vi "test - Unregister Status Registration.vi"(8 "error in (no error)":errorcluster, 11 "TestCase in":refnum<class "testcase-Broadcast Registry.lvclass">) -> (0 "error out":errorcluster, 3 "TestCase out":refnum<class "testcase-Broadcast Registry.lvclass">)   [LabVIEW 2017, in "testcase-Broadcast Registry.lvclass"]
uses:
  testcase-Broadcast Registry.lvclass
  f1ab6f25-c30d-499f-96ca-3a55fa643449.vi
  src/user.lib/_NEVSTOP/Communicable State Machine(CSM)/AdvanceAPI/CSM - Revert Arguments-Safe String.vi
  src/user.lib/_NEVSTOP/Communicable State Machine(CSM)/AdvanceAPI/CSM - Make String Arguments Safe.vi
  src/user.lib/_NEVSTOP/Communicable State Machine(CSM)/AdvanceAPI/CSM - Break Down Multiple States String.vi
  src/user.lib/_NEVSTOP/Communicable State Machine(CSM)/AdvanceAPI/CSM - Compact Multiple States.vi
  src/user.lib/_NEVSTOP/Communicable State Machine(CSM)/AdvanceAPI/CSM - Keywords.vi
  src/user.lib/_NEVSTOP/Communicable State Machine(CSM)/_Shared/Trim Single-line Text.vi
  <vilib>/addons/_JKI Toolkits/VI Tester/TestCase.llb/TestCase.lvclass
  src/user.lib/_NEVSTOP/Communicable State Machine(CSM)/Communicable State Machine.lvlib
  C:/Program Files (x86)/National Instruments/LabVIEW 2017/vi.lib/addons/_JKI Toolkits/VI Tester/TestCase.llb/TestCase.lvclass
panel:
  out "Entries":T1(array[cluster])
  out "Error Occurred":errorcluster
  out "State History":string
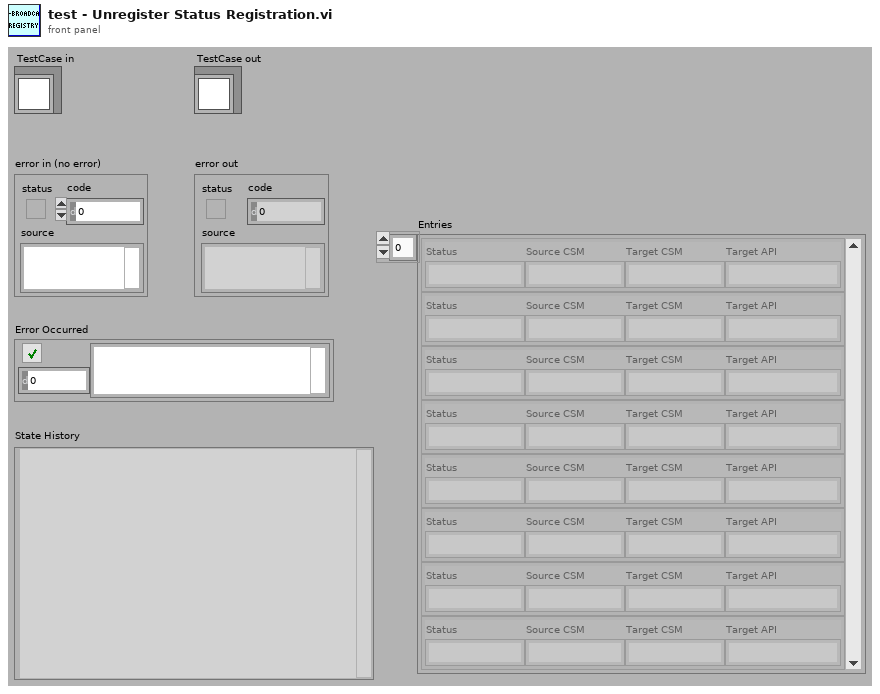
[diagram p1: front panel]
types:
  T1 = cluster{"Status":string, "Source CSM":string, "Target CSM":string, "Target API":string}[]
  T2 = enum32{"Invalid", "Standard", "Closed", "Hidden", "Minimized", "Maximized"}
  T3 = enum32{"invalid app kind", "Development System", "Run Time System", "Student Edition", "Embedded LabVIEW", "Evaluation", "Custom"}
  T4 = typedef "Communicable State Machine.lvlib/_CSM_Response Source Message.ctl" = cluster{"‘State":string, "’Arguments":string, "’Error":errorcluster}
  T5 = cluster{"Current VI Reference":refnum<vi>, "Close Panel on Exit?":bool}
  T6 = cluster{"Core":cluster{"Current VI Reference":refnum<vi>, "Close Panel on Exit?":bool}, "Your Boolean data":bool, "Your string data":string}
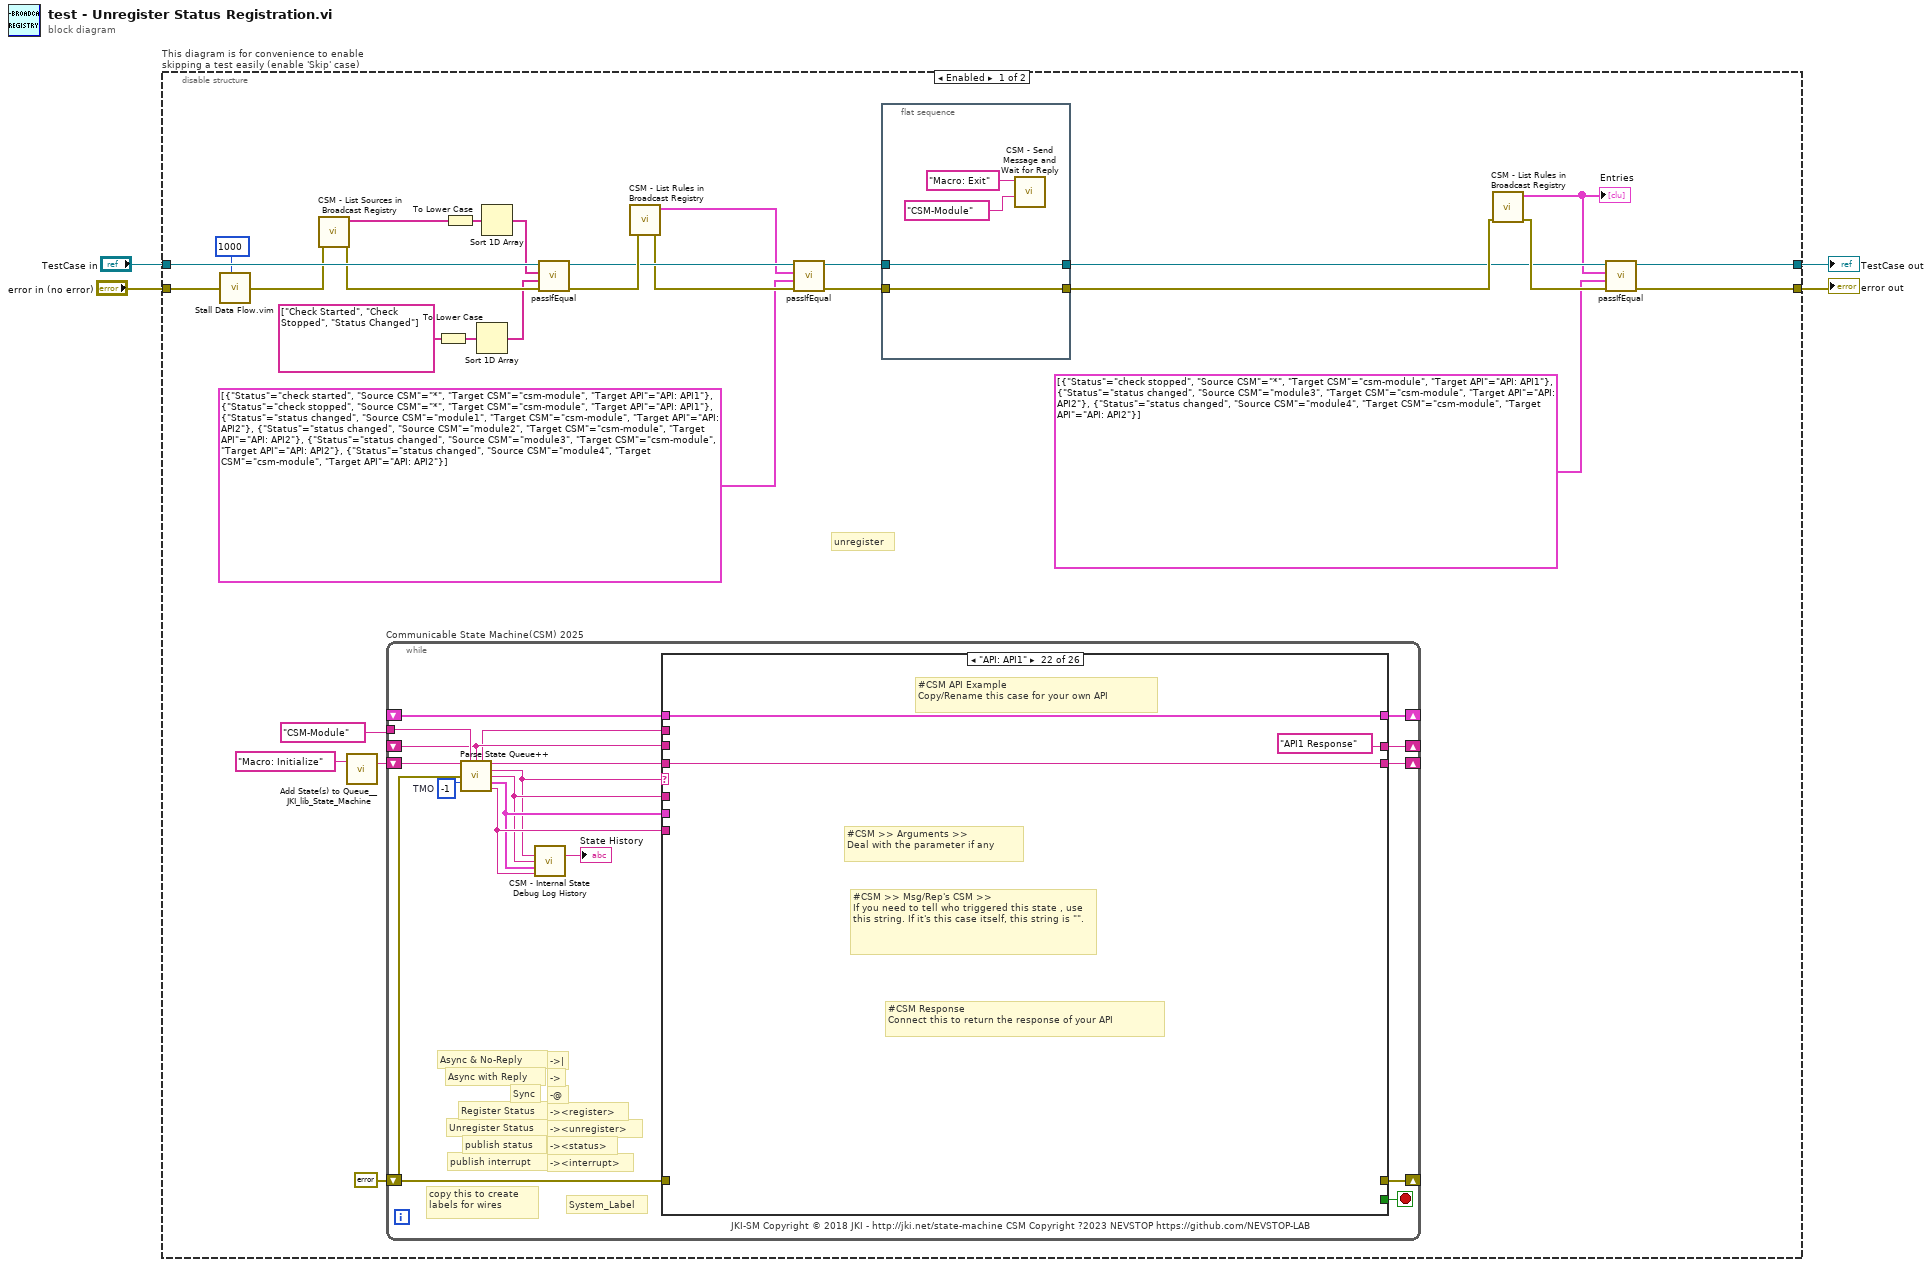
[diagram p0: block diagram]
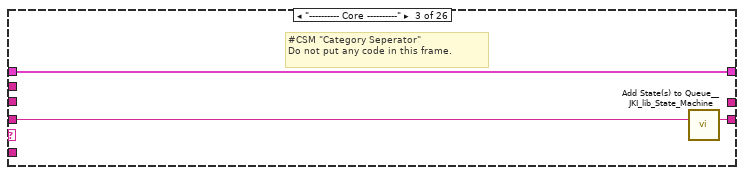
[diagram p4: hidden frame]
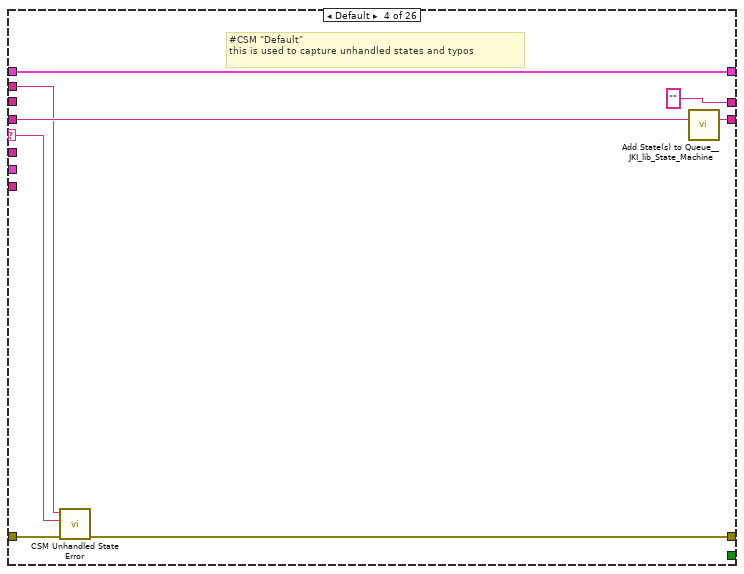
[diagram p5: hidden frame]
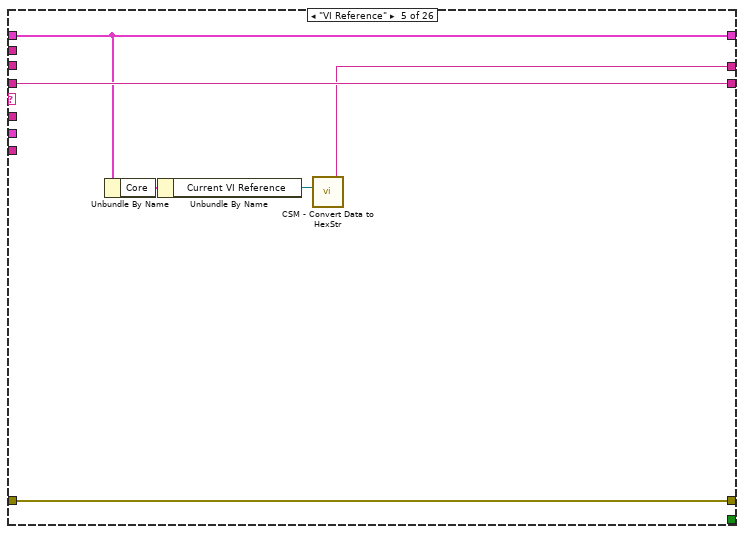
[diagram p6: hidden frame]
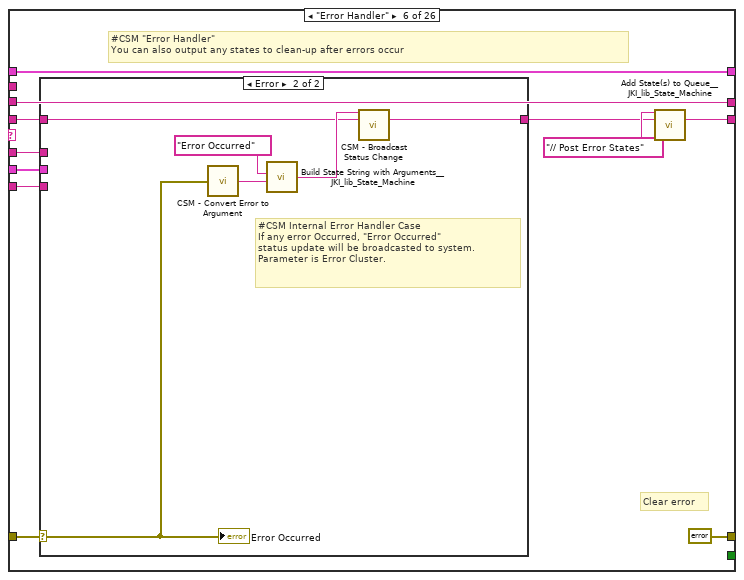
[diagram p7: hidden frame]
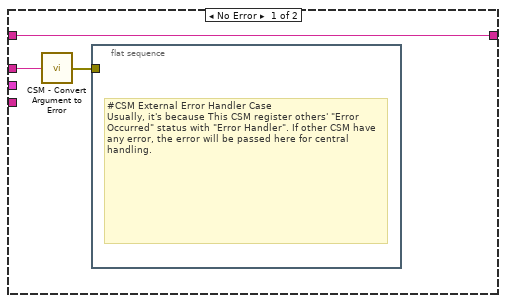
[diagram p8: hidden frame]
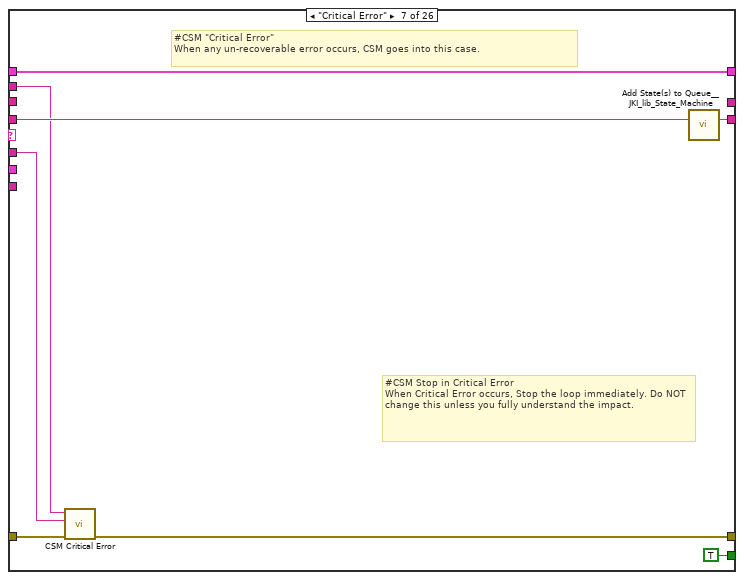
[diagram p9: hidden frame]
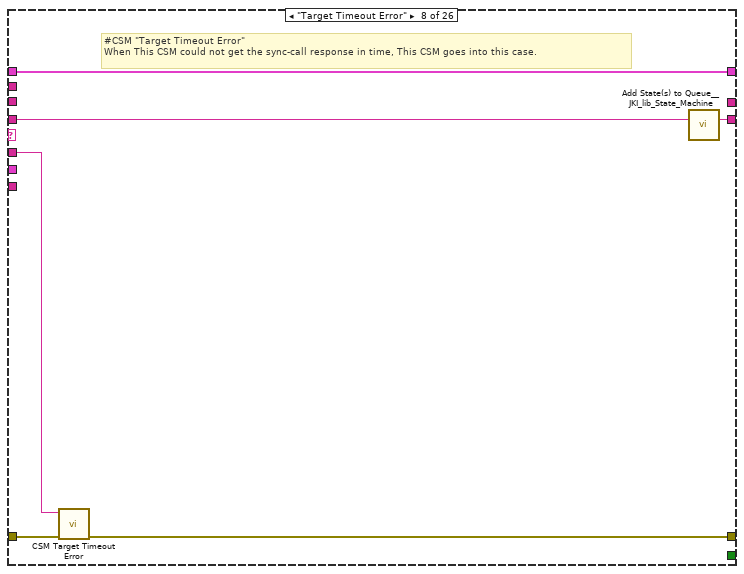
[diagram p10: hidden frame]
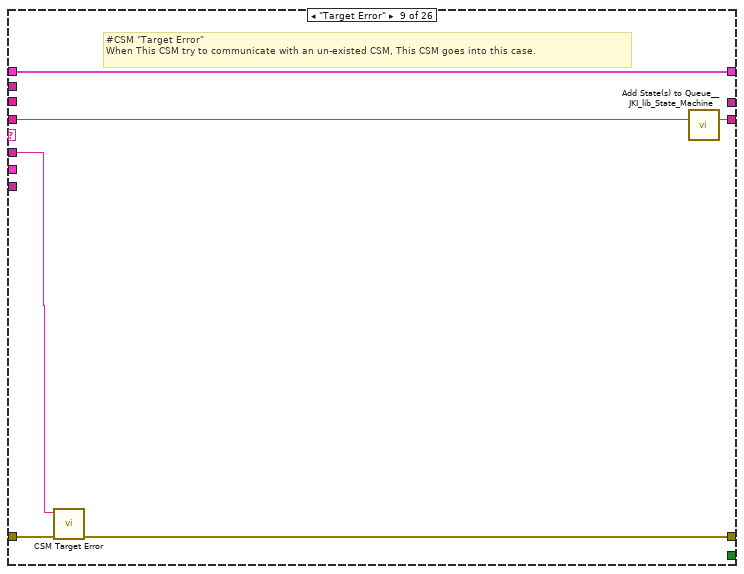
[diagram p11: hidden frame]
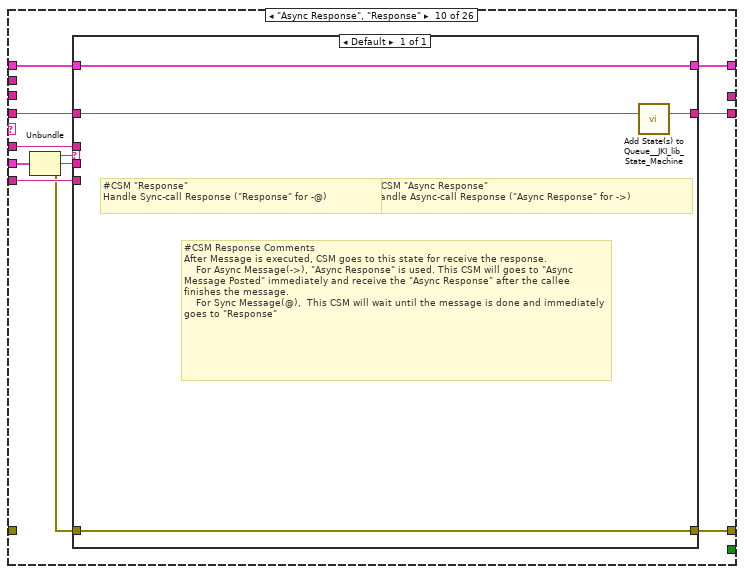
[diagram p12: hidden frame]
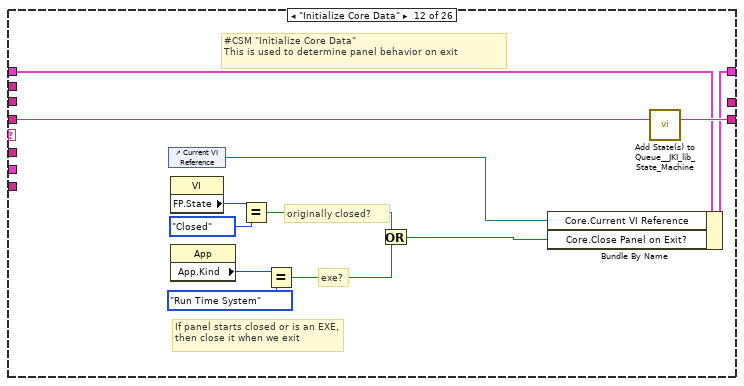
[diagram p14: hidden frame]
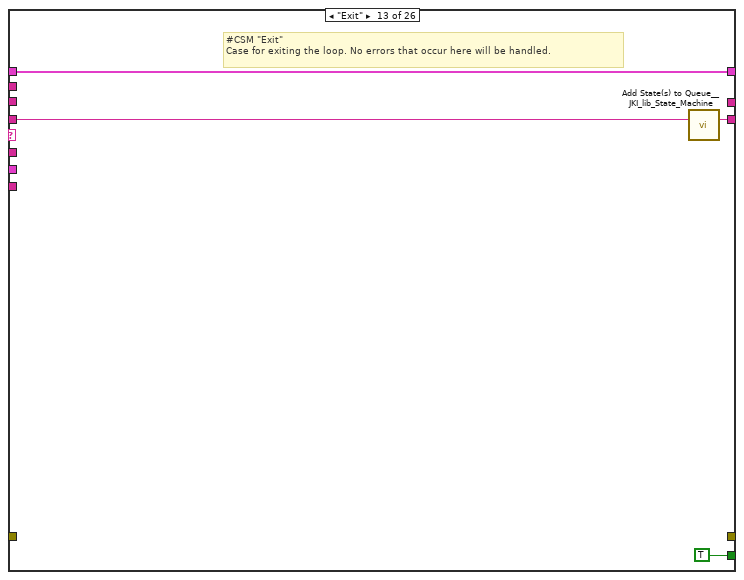
[diagram p15: hidden frame]
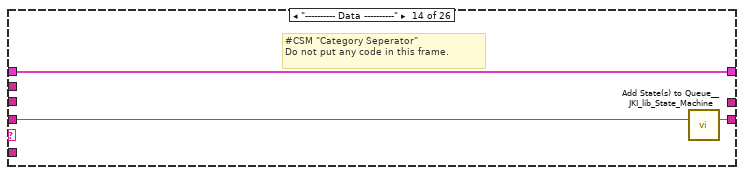
[diagram p16: hidden frame]
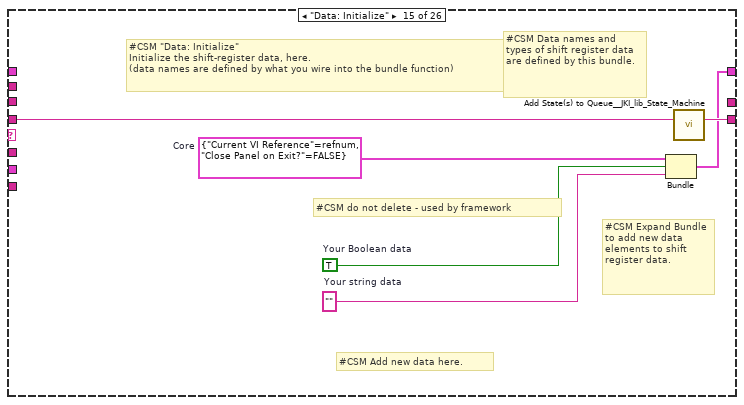
[diagram p17: hidden frame]
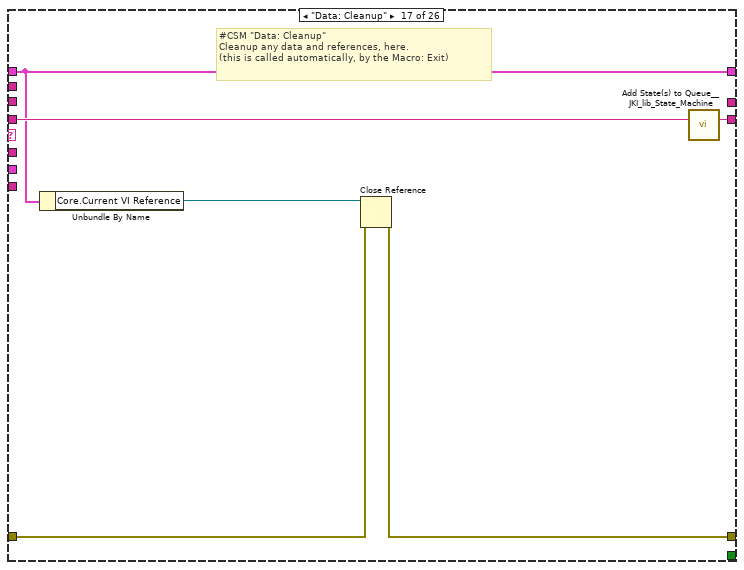
[diagram p19: hidden frame]
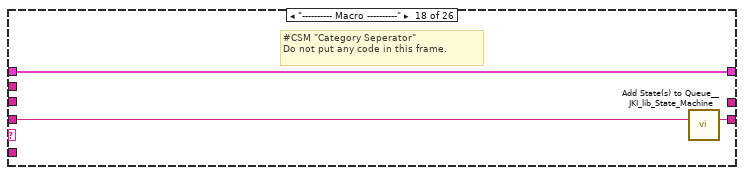
[diagram p20: hidden frame]
diagram:
  n1 = disable-structure "This diagram is for convenience to enable skipping a test easily (enable 'Skip' case)" shown="Enabled" {
    disable-tunnel: "TestCase in" -> [w33 w203]
    disable-tunnel: [w8 w201] -> w1
    disable-tunnel: [w7 w202] -> w3
    disable-tunnel: "error in (no error)" -> [w32 w200]
    frame Enabled {
      # "unregister"
      n2 = call "Stall Data Flow.vim"("value in"=w32, "milliseconds to wait"=u32 1000) -> ("value out"=w27:errorcluster)  [unwired: 1 out]
      n3 = call "CSM - List Sources in Broadcast Registry.vi"("error in (no error)"=w27) -> ("error out"=w25:errorcluster, "Broadcast Names"=w24:string[])  [unwired: 9 in]
      n4 = call <vilib>:"Add State(s) to Queue__JKI_lib_State_Machine.vi"("State(s) in (\"\")"="Macro: Initialize" ("Init State(\"Macro: Initialize\")")) -> ("States Out"=w31:string)  [unwired: 14 in]
      n5 = while "Communicable State Machine(CSM) 2025" {
        shift-right: [w50] -> _
        shift-left: _ -> [w49]
        shift-right: [w53] -> _
        shift-left: errorcluster {"status"=FALSE, "code"=0, "source"=""} ("error out") -> [w39]
        shift-right: [w52] -> _
        shift-left: w31 -> [w54]
        tunnel: "CSM-Module" ("Name (\"\" to Use UUID)") -> [w46]
        shift-right: [w47] -> _
        shift-left: _ -> [w41]
        stop <- w51 stop-if-true
        w48 = -1  # TMO
        # "-><interrupt>"
        # "-><status>"
        # "-><unregister>"
        # "-><register>"
        # "-@"
        # "->"
        # "->|"
        # "publish interrupt"
        # "publish status"
        # "Unregister Status"
        # "Register Status"
        # "Sync"
        # "Async with Reply"
        # "Async & No-Reply"
        # "JKI-SM Copyright © 2018 JKI - http://jki.net/state-machine CSM Copyright ?2023 NEVSTOP https://github.com/NEVSTOP-LAB"
        # "copy this to create labels for wires"
        # "System_Label"
        n6 = call "Parse State Queue++.vi"("State Queue"=w54, "Name (\"\" to Use UUID)"=w46, "Response Arguments"=w41, "Previous Error"=w39, "Dequeue (1 ms)"=w48) -> ("Name Used"=w40:string, "Remaining States"=w55:string, "Current State"=w42:string, "Arguments"=w43:string, "Additional Information"=w44:T4, "Source CSM"=w45:string)  [unwired: 5 in]
        n7 = call "CSM - Internal State Debug Log History.vi"("State"=w42, "Arguments (\"\")"=w43, ">> Response Source Message >>"=w44, "Source (\"\")"=w45) -> ("Debug Log"=→"State History":string)  [unwired: 11 in]
        n8 = case shown="\"API: API1\"" w42 {
          selector: w42 -> [_ _ _ w66 _ _ _ _ _ _ _ _ _ _ _ _ _ _ _ _ _ _ _ _ _ _]
          tunnel: w55 -> [w56 w59 w62 w70 w75 w81 w104 w110 w116 w126 w133 w145 w149 w152 w158 w160 w166 w169 w173 w179 w181 w184 w188 w193 w196 w199]
          tunnel: w43 -> [_ _ _ _ _ w80 w100 w107 w113 w120 _ _ _ _ _ _ _ _ _ _ _ _ w186 _ _ _]
          tunnel: w49 -> [w57 w58 w60 w68 w74 w86 w102 w108 w114 w124 w132 w139 w147 w150 _ w159 w161 w167 w171 w177 w180 w183 w187 w191 w194 w197]
          tunnel: [_ _ _ w63 w76 errorcluster {"status"=FALSE, "code"=0, "source"=""} ("error out") w97 w105 w111 w127 _ _ _ _ _ _ w162 _ _ _ _ _ _ _ _ _] -> w53
          tunnel: w39 -> [_ _ _ w64 w76 w84 w98 w106 w112 _ _ _ _ _ _ _ w163 _ _ _ _ _ _ _ _ _]
          tunnel: [w56 w59 w61 w69 w75 w82 w103 w109 w115 w125 w133 w144 w148 w151 w157 w160 w165 w168 w172 w178 w181 w184 w188 w192 w195 w198] -> w52
          tunnel: [_ _ _ _ _ _ TRUE _ _ _ _ _ TRUE _ _ _ _ _ _ _ _ _ _ _ _ _] -> w51
          tunnel: [w57 w58 w60 w68 w74 w86 w102 w108 w114 w123 w132 w143 w147 w150 w156 w159 w161 w167 w171 w177 w180 w183 w187 w191 w194 w197] -> w50
          tunnel: w45 -> [_ _ _ _ _ w79 _ _ _ w121 _ _ _ _ _ _ _ _ _ _ _ _ _ _ _ _]
          tunnel: w44 -> [_ _ _ _ _ w78 _ _ _ w122 _ _ _ _ _ _ _ _ _ _ _ _ _ _ _ _]
          tunnel: [_ _ _ "" w71 w77 _ _ _ _ _ _ _ _ _ _ _ _ _ _ _ "API1 Response" w185 _ _ _] -> w47
          tunnel: w40 -> [_ _ _ w65 _ _ w99 _ _ _ _ _ _ _ _ _ _ _ _ _ _ _ _ _ _ _]
          tunnel: w41 -> [_ _ _ _ _ w77 _ _ _ _ _ _ _ _ _ _ _ _ _ _ _ _ _ _ _ _]
          frame "", "Idle" {
            # "#CSM \"Idle/Event Handler\"\nexecutes when the state queue is empty"
          }
          frame "CSM Documentation" {
            # "#CSM Documentation"
            # "#CSM State Syntax\n\n// Comment line, all text to the right of “//” will be ignored\n// Local Message Example\nDoSth: DoA >> Arguments\n\n// Sync Call Example\nAPI: xxxx >> Arguments -@ TargetModule\n\n// Async Call Example\nAPI: xxxx >> Arguments -> TargetModule\n\n// Async Call without Reply Example\nAPI: xxxx >> Arguments ->| TargetModule\n\n// Broadcast normal status:\nStatus >> StatusArguments  -><status>\n\n// Broadcast Interrupt status:\nInterrupt >> StatusArguments  -><interrupt>\n\n// Register Source Module's status to Handler Module\nStatus@Source Module >> Handler Module@Handler Module -><register>\n\n// Unegister Source Module's status\nStatus@Source Module >> Handler Module -><unregister>"
            # "#CSM README FIRST\n\nCommunicable State Machine(CSM) is a LabVIEW application framework that builds upon JKI State Machine(JKISM). It follows the pattern of JKISM and extends the keywords to describe message communication between modules, including concepts such as Sync-Message, Async-Message, Subscription/Unsubscription of status - essential elements for creating reusable code modules. For more information, please visit the CSM wiki: https://nevstop-lab.github.io/CSM-Wiki/\n\nFor instructions on JKI State Machine, visit: \n    http://jki.net/state-machine/\nFor information about CSM, visit: \n    https://github.com/NEVSTOP-LAB"
            # "#CSM \"Documentation\"\nCase for holding CSM Documenation"
          }
          frame "---------- Core ----------" {
            # "#CSM \"Category Seperator\"\nDo not put any code in this frame."
            n9 = call <vilib>:"Add State(s) to Queue__JKI_lib_State_Machine.vi"("State(s) in (\"\")"=w62) -> ("States Out"=w61:string)  [unwired: 14 in]
          }
          frame Default {
            # "#CSM \"Default\"\nthis is used to capture unhandled states and typos"
            n10 = call "CSM Unhandled State Error.vi"("error in (no error)"=w64, "Undefined State"=w66, "CSM Name"=w65) -> ("error out"=w63:errorcluster)  [unwired: 8 in]
            n11 = call <vilib>:"Add State(s) to Queue__JKI_lib_State_Machine.vi"("State(s) in (\"\")"=w70) -> ("States Out"=w69:string)  [unwired: 14 in]
          }
          frame "VI Reference" {
            n12 = Unbundle By Name(w74) -> ("Core"=w73:T5)
            n13 = Unbundle By Name(w73) -> ("Current VI Reference"=w72:refnum<vi>)
            n14 = call "CSM - Convert Data to HexStr.vi"("Variant"=w72) -> ("HEX String (0-9,A-F)"=w71:string)  [unwired: 8 in]
          }
          frame "Error Handler" {
            # "#CSM \"Error Handler\"\nYou can also output any states to clean-up after errors occur"
            # "Clear error"
            n15 = case shown="Error" w84 {
              selector: w84 -> [_ w91]
              tunnel: [w90 w93] -> w83
              tunnel: w81 -> [w90 w92]
              tunnel: w80 -> [w89 _]
              tunnel: w79 -> [_ _]
              tunnel: w78 -> [_ _]
              frame No Error {
                n16 = call "CSM - Convert Argument to Error.vi"("Argument"=w89) -> ("Error"=w88:errorcluster)  [unwired: 4 in]
                n17 = flat-sequence {
                  tunnel: w88 -> [_]
                  frame #0 {
                    # "#CSM External Error Handler Case\nUsually, it's because This CSM register others' \"Error Occurred\" status with \"Error Handler\". If other CSM have any error, the error will be passed here for central handling."
                  }
                }
              }
              frame Error {
                # "#CSM Internal Error Handler Case \nIf any error Occurred, \"Error Occurred\" \nstatus update will be broadcasted to system.\nParameter is Error Cluster."
                n18 = call "CSM - Convert Error to Argument.vi"("Error"=w91) -> ("Argument"=w95:string)  [unwired: 4 in]
                n19 = call <vilib>:"Build State String with Arguments__JKI_lib_State_Machine.vi"("Arguments (\"\")"=w95, "State"="Error Occurred" ("Status with Arguments")) -> ("State with Arguments"=w94:string)  [unwired: 4 in]
                n20 = call "CSM - Broadcast Status Change.vi"("Status With Arguments"=w94, "State Queue"=w92) -> ("Remaining States"=w93:string)  [unwired: 13 in]
                "Error Occurred" <- w91
              }
            }
            n21 = call <vilib>:"Add State(s) to Queue__JKI_lib_State_Machine.vi"("State(s) in Front (\"\")"="// Post Error States", "State(s) in (\"\")"=w83) -> ("States Out"=w82:string)  [unwired: 13 in]
          }
          frame "Critical Error" {
            # "#CSM \"Critical Error\"\nWhen any un-recoverable error occurs, CSM goes into this case."
            # "#CSM Stop in Critical Error\nWhen Critical Error occurs, Stop the loop immediately. Do NOT change this unless you fully understand the impact."
            n22 = call "CSM Critical Error.vi"("error in (no error)"=w98, "Arugments (As Reason)"=w100, "CSM Name"=w99) -> ("error out"=w97:errorcluster)  [unwired: 8 in]
            n23 = call <vilib>:"Add State(s) to Queue__JKI_lib_State_Machine.vi"("State(s) in (\"\")"=w104) -> ("States Out"=w103:string)  [unwired: 14 in]
          }
          frame "Target Timeout Error" {
            # "#CSM \"Target Timeout Error\"\nWhen This CSM could not get the sync-call response in time, This CSM goes into this case."
            n24 = call "CSM Target Timeout Error.vi"("error in (no error)"=w106, "Arguments (As CSM Name)"=w107) -> ("error out"=w105:errorcluster)  [unwired: 9 in]
            n25 = call <vilib>:"Add State(s) to Queue__JKI_lib_State_Machine.vi"("State(s) in (\"\")"=w110) -> ("States Out"=w109:string)  [unwired: 14 in]
          }
          frame "Target Error" {
            # "#CSM \"Target Error\"\nWhen This CSM try to communicate with an un-existed CSM, This CSM goes into this case."
            n26 = call "CSM Target Error.vi"("error in (no error)"=w112, "Arguments (As CSM Name)"=w113) -> ("error out"=w111:errorcluster)  [unwired: 9 in]
            n27 = call <vilib>:"Add State(s) to Queue__JKI_lib_State_Machine.vi"("State(s) in (\"\")"=w116) -> ("States Out"=w115:string)  [unwired: 14 in]
          }
          frame "Async Response", "Response" {
            n28 = Unbundle(w122) -> ("‘State"=w119:string, "’Arguments"=w118:string, "’Error"=w117:errorcluster)
            n29 = case shown="Default" w119 {
              tunnel: [w128] -> w125
              tunnel: w126 -> [w129]
              tunnel: [w131] -> w123
              tunnel: w124 -> [w131]
              tunnel: [w130] -> w127
              tunnel: w117 -> [w130]
              tunnel: w121 -> [_]
              tunnel: w120 -> [_]
              tunnel: w118 -> [_]
              frame Default {
                # "#CSM \"Async Response\"\nHandle Async-call Response (\"Async Response\" for ->)"
                # "#CSM \"Response\"\nHandle Sync-call Response (\"Response\" for -@)"
                # "#CSM Response Comments\nAfter Message is executed, CSM goes to this state for receive the response.\n    For Async Message(->), \"Async Response\" is used. This CSM will goes to \"Async Message Posted\" immediately and receive the \"Async Response\" after the callee finishes the message.\n    For Sync Message(@),  This CSM will wait until the message is done and immediately goes to \"Response\""
                n30 = call <vilib>:"Add State(s) to Queue__JKI_lib_State_Machine.vi"("State(s) in (\"\")"=w129) -> ("States Out"=w128:string)  [unwired: 14 in]
              }
            }
          }
          frame "Async Message Posted" {
            # "#CSM \"Async Message Posted\"\nAfter Async Message is posted (-> or ->| ), CSM goes to this state for post-action.\nYou can use Argument - State to tell which Async Message is called."
          }
          frame "Initialize Core Data" {
            # "#CSM \"Initialize Core Data\"\nThis is used to determine panel behavior on exit"
            # "originally closed?"
            # "exe?"
            # "If panel starts closed or is an EXE, then close it when we exit"
            n31 = control-ref of="Current VI Reference"() -> (w137:refnum<vi>)
            n32 = property class="VI"() -> ("FP.State"=w136:T2)  [unwired: 2 in, 2 out]
            n33 = property class="App"() -> ("App.Kind"=w142:T3)  [unwired: 2 in, 2 out]
            n34 = Equal?(x=w136, y=T2."Closed" ("Front Panel Window:State")) -> (x = y?=w134:bool)
            n35 = Equal?(x=w142, y=T3."Run Time System" ("Application:Kind")) -> (x = y?=w140:bool)
            n36 = Or(x=w134, y=w140) -> (x .or. y?=w138:bool)
            n37 = Bundle By Name(cluster=w139, "Core.Current VI Reference"=w137, "Core.Close Panel on Exit?"=w138) -> (w143:T6)
            n38 = call <vilib>:"Add State(s) to Queue__JKI_lib_State_Machine.vi"("State(s) in (\"\")"=w145) -> ("States Out"=w144:string)  [unwired: 14 in]
          }
          frame "Exit" {
            # "#CSM \"Exit\"\nCase for exiting the loop. No errors that occur here will be handled."
            n39 = call <vilib>:"Add State(s) to Queue__JKI_lib_State_Machine.vi"("State(s) in (\"\")"=w149) -> ("States Out"=w148:string)  [unwired: 14 in]
          }
          frame "---------- Data ----------" {
            # "#CSM \"Category Seperator\"\nDo not put any code in this frame."
            n40 = call <vilib>:"Add State(s) to Queue__JKI_lib_State_Machine.vi"("State(s) in (\"\")"=w152) -> ("States Out"=w151:string)  [unwired: 14 in]
          }
          frame "Data: Initialize" {
            w153 = T5 {"Current VI Reference"=refnum, "Close Panel on Exit?"=FALSE}  # Core
            w155 = TRUE  # Your Boolean data
            w154 = ""  # Your string data
            # "#CSM \"Data: Initialize\"\nInitialize the shift-register data, here.\n(data names are defined by what you wire into the bundle function)"
            # "#CSM do not delete - used by framework"
            # "#CSM Expand Bundle to add new data elements to shift register data."
            # "#CSM Add new data here."
            # "#CSM Data names and types of shift register data are defined by this bundle."
            n41 = Bundle("Core"=w153, "Your Boolean data"=w155, "Your string data"=w154) -> (w156:T6)  [unwired: 1 in]
            n42 = call <vilib>:"Add State(s) to Queue__JKI_lib_State_Machine.vi"("State(s) in (\"\")"=w158) -> ("States Out"=w157:string)  [unwired: 14 in]
          }
          frame "Data: Update Indicators" {
          }
          frame "Data: Cleanup" {
            # "#CSM \"Data: Cleanup\"\nCleanup any data and references, here.\n(this is called automatically, by the Macro: Exit)"
            n43 = Unbundle By Name(w161) -> ("Core.Current VI Reference"=w164:refnum<vi>)
            n44 = Close Reference(reference=w164, error in (no error)=w163) -> (error out=w162:errorcluster)
            n45 = call <vilib>:"Add State(s) to Queue__JKI_lib_State_Machine.vi"("State(s) in (\"\")"=w166) -> ("States Out"=w165:string)  [unwired: 14 in]
          }
          frame "---------- Macro ----------" {
            # "#CSM \"Category Seperator\"\nDo not put any code in this frame."
            n46 = call <vilib>:"Add State(s) to Queue__JKI_lib_State_Machine.vi"("State(s) in (\"\")"=w169) -> ("States Out"=w168:string)  [unwired: 14 in]
          }
          frame "Macro: Initialize" {
            # "#CSM \"Macro: Initialize\"\nInitialization Macro (This is called once, when the VI starts)"
            n47 = call <vilib>:"Add State(s) to Queue__JKI_lib_State_Machine.vi"("State(s) in Front (\"\")"="Data: Initialize\nInitialize Core Data\nData: Update Indicators\nCheck Started@* >> API: API1 -><register>\nCheck Stopped@* >> API: API1@CSM-Module -><register>\nStatus Changed@module1 >> API: API2 -><register>\nStatus Changed@module2 >> API: API2 -><register>\nStatus Changed@module3 >> API: API2@CSM-Module -><register>\nStatus Changed@module4 >> API: API2@CSM-Module -><register>", "State(s) in (\"\")"=w173) -> ("States Out"=w172:string)  [unwired: 13 in]
          }
          frame "Macro: Exit" {
            # "#CSM \"Macro: Exit\"\nExit Macro (This is called once, when the VI exits)"
            n48 = call <vilib>:"Add State(s) to Queue__JKI_lib_State_Machine.vi"("State(s) in Front (\"\")"="//Exit Sub-Modules ", "State(s) at Back (\"\")"="Check Started@* -><unregister>\nStatus Changed@module1  -><unregister>\nStatus Changed@module2  -><unregister>\nData: Cleanup\nExit") -> ("States Out"=w175:string)  [unwired: 13 in]
            n49 = call <vilib>:"Add State(s) to Queue__JKI_lib_State_Machine.vi"("State(s) in Front (\"\")"=w175, "State(s) in (\"\")"=w179) -> ("States Out"=w178:string)  [unwired: 13 in]
          }
          frame "---------- API ----------" {
            # "#CSM \"Category Seperator\"\nDo not put any code in this frame."
          }
          frame "API: API1" {
            # "#CSM API Example\nCopy/Rename this case for your own API"
            # "#CSM >> Msg/Rep's CSM >>\nIf you need to tell who triggered this state , use this string. If it's this case itself, this string is \"\"."
            # "#CSM >> Arguments >>\nDeal with the parameter if any"
            # "#CSM Response\nConnect this to return the response of your API"
          }
          frame "API: API2" {
            # "#CSM API Example\nCopy/Rename this case for your own API"
            # "unpack Hex String  to Variant\nif complex parameter is needed."
            n50 = call "CSM - Convert HexStr to Data.vi"("HEX String"=w186) -> ()  [unwired: 7 in, 2 out]
            n51 = disable-structure shown="Disabled" {
              disable-tunnel: [w189 "API2 Response"] -> w185
              frame Disabled {
                # "pack variant to hexstr \nif complex response is needed."
                # "complex Response"
                n52 = call "CSM - Convert Data to HexStr.vi"() -> ("HEX String (0-9,A-F)"=w189:string)  [unwired: 9 in]
              }
              frame Enabled {
              }
            }
          }
          frame "---------- Action ----------" {
            # "#CSM \"Category Seperator\"\nDo not put any code in this frame."
            n53 = call <vilib>:"Add State(s) to Queue__JKI_lib_State_Machine.vi"("State(s) in (\"\")"=w193) -> ("States Out"=w192:string)  [unwired: 14 in]
          }
          frame "Action: action1" {
            # "#CSM \"Internal State\"\nThis category is used for holding internal states"
            n54 = call <vilib>:"Add State(s) to Queue__JKI_lib_State_Machine.vi"("State(s) in (\"\")"=w196) -> ("States Out"=w195:string)  [unwired: 14 in]
          }
          frame "Action: action2" {
            # "#CSM \"Internal State\"\nThis category is used for holding internal states"
            n55 = call <vilib>:"Add State(s) to Queue__JKI_lib_State_Machine.vi"("State(s) in (\"\")"=w199) -> ("States Out"=w198:string)  [unwired: 14 in]
          }
        }
      }
      n56 = To Lower Case(string=string[] ["Check Started", "Check Stopped", "Status Changed"] ("Status in Registry")) -> (all lower case string=w20:string[])
      n57 = To Lower Case(string=w24) -> (all lower case string=w19:string[])
      n58 = Sort 1D Array(array=w20) -> (sorted array=w21:string[])
      n59 = Sort 1D Array(array=w19) -> (sorted array=w22:string[])
      n60 = call-dynamic "passIfEqual.vi"("error in (no error)"=w25, "y"=w21, "x"=w22, "TestCase in"=w33) -> ("error out"=w18:errorcluster, "TestCase out"=w17:refnum<class "testcase-Broadcast Registry.lvclass">)  [unwired: 6 in]
      n61 = call "CSM - List Rules in Broadcast Registry.vi"("error in (no error)"=w18) -> ("error out"=w16:errorcluster, "Rule Entries"=w14:T1)  [unwired: 9 in]
      n62 = call-dynamic "passIfEqual.vi"("error in (no error)"=w16, "y"=T1 [{"Status"="check started", "Source CSM"="*", "Target CSM"="csm-module", "Target API"="API: API1"}, {"Status"="check stopped", "Source CSM"="*", "Target CSM"="csm-module", "Target API"="API: API1"}, {"Status"="status changed", "Source CSM"="module1", "Target CSM"="csm-module", "Target API"="API: API2"}, {"Status"="status changed", "Source CSM"="module2", "Target CSM"="csm-module", "Target API"="API: API2"}, {"Status"="status changed", "Source CSM"="module3", "Target CSM"="csm-module", "Target API"="API: API2"}, {"Status"="status changed", "Source CSM"="module4", "Target CSM"="csm-module", "Target API"="API: API2"}] ("Entries"), "x"=w14, "TestCase in"=w17) -> ("error out"=w15:errorcluster, "TestCase out"=w13:refnum<class "testcase-Broadcast Registry.lvclass">)  [unwired: 6 in]
      n63 = flat-sequence {
        tunnel: [w35] -> w11
        tunnel: w15 -> [w35]
        tunnel: [w34] -> w9
        tunnel: w13 -> [w34]
        frame #0 {
          n64 = call "CSM - Send Message and Wait for Reply.vi"("Target Module"="CSM-Module" ("Name (\"\" to Use UUID)"), "State"="Macro: Exit") -> ()  [unwired: 7 in, 3 out]
        }
      }
      n65 = call "CSM - List Rules in Broadcast Registry.vi"("error in (no error)"=w11) -> ("error out"=w10:errorcluster, "Rule Entries"=w6:T1)  [unwired: 9 in]
      "Entries" <- w6
      n66 = call-dynamic "passIfEqual.vi"("error in (no error)"=w10, "y"=T1 [{"Status"="check stopped", "Source CSM"="*", "Target CSM"="csm-module", "Target API"="API: API1"}, {"Status"="status changed", "Source CSM"="module3", "Target CSM"="csm-module", "Target API"="API: API2"}, {"Status"="status changed", "Source CSM"="module4", "Target CSM"="csm-module", "Target API"="API: API2"}] ("Entries"), "x"=w6, "TestCase in"=w9) -> ("error out"=w7:errorcluster, "TestCase out"=w8:refnum<class "testcase-Broadcast Registry.lvclass">)  [unwired: 6 in]
    }
    frame Disabled {
      # "skip test result while test is under development"
      n67 = call <vilib>:"skip.vi"("error in (no error)"=w200, "TestCase in"=w203) -> ("error out"=w202:errorcluster, "TestCase out"=w201:refnum<class "testcase-Broadcast Registry.lvclass">)  [unwired: 8 in]
    }
  }
  "error out" <- w3
  "TestCase out" <- w1
